vi "TIO Data Stream Flatten.vi"(1 "Data Out":T1(array[cluster])=[{"Name"="gmr", "Waveform"={"start"=0.0, "dt"=1.0, "Timeseries"=[[-1045203.6, 2103369.2, -524451.06]]}}, {"Name"="accel", "Waveform"={"start"=0.0, "dt"=1.0, "Timeseries"=[[0.4673273, -9.214466, -3.0972874]]}}, {"Name"="gyro", "Waveform"={"start"=0.0, "dt"=1.0, "Timeseries"=[[0.019417262, 0.008815161, 0.006293709]]}}, {"Name"="bar", "Waveform"={"start"=0.0, "dt"=1.0, "Timeseries"=[[0.0]]}}, {"Name"="therm", "Waveform"={"start"=0.0, "dt"=1.0, "Timeseries"=[[0.0]]}}]) -> (0 "Flattened Array":sgl[][](array[numeric]))   [LabVIEW 2010]
panel:
  # "TIO Data Stream Flatten to Array"
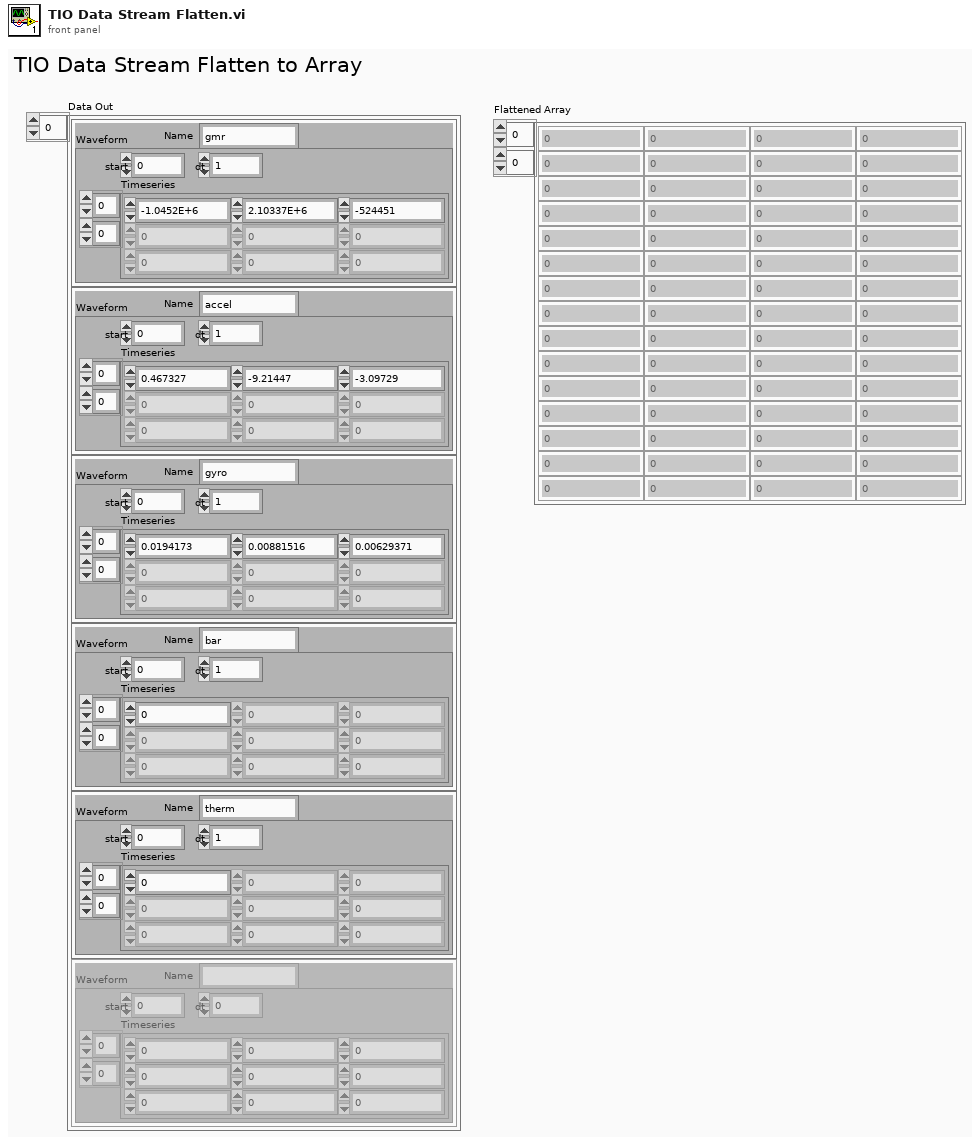
[diagram p1: front panel]
types:
  T1 = cluster{"Name":string, "Waveform":cluster{"start":dbl, "dt":dbl, "Timeseries":sgl[][]}}[]
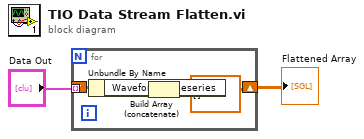
[diagram p0: block diagram]
diagram:
  n1 = for {
    tunnel: "Data Out" -> [w7] mode=indexing
    shift-right: [w4] -> w2
    shift-left: sgl[][] [] ("Timeseries") -> [w5]
    n2 = Unbundle By Name(w7) -> ("Waveform.Timeseries"=w6:sgl[][])
    n3 = Build Array (concatenate)(w5, w6) -> (w4:sgl[][])
  }
  "Flattened Array" <- w2
